vi "POST (Multipart).vi"(6 "timeout":i32=10000, 7 "output file":path, 8 "error in":errorcluster, 9 "data":T1[](array[typedef]), 10 "url":string, 11 "Session In":refnum<class "Session.lvclass">) -> (0 "error out":errorcluster, 1 "body":string, 2 "headers":string, 3 "Session Out":refnum<class "Session.lvclass">, 4 "status code":u32)   [LabVIEW 2020, in "Library Commun.lvlib" / "Library Http.lvlib" / "Session.lvclass"]
uses:
  Session.lvclass
  Multipart Data--cluster.ctl
  Session.lvclass/Session.ctl
  lvwebclient_32.dll
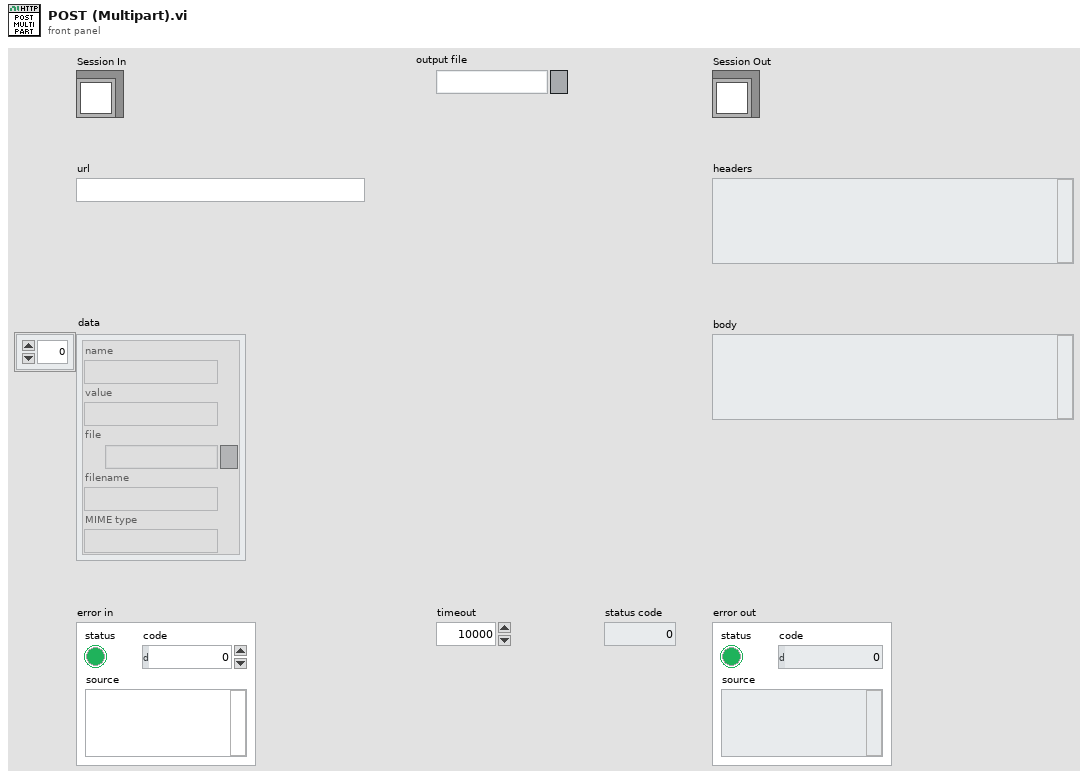
[diagram p1: front panel]
types:
  T1 = typedef "Library Commun.lvlib/Library Http.lvlib/Session.lvclass/Multipart Data--cluster.ctl" = cluster{"name":string, "value":string, "file":path, "filename":string, "MIME type":string}
  T2 = cluster{"utf-8 text":string, "utf-8 text":string, "file":path, "utf-8 text":string, "utf-8 text":string}
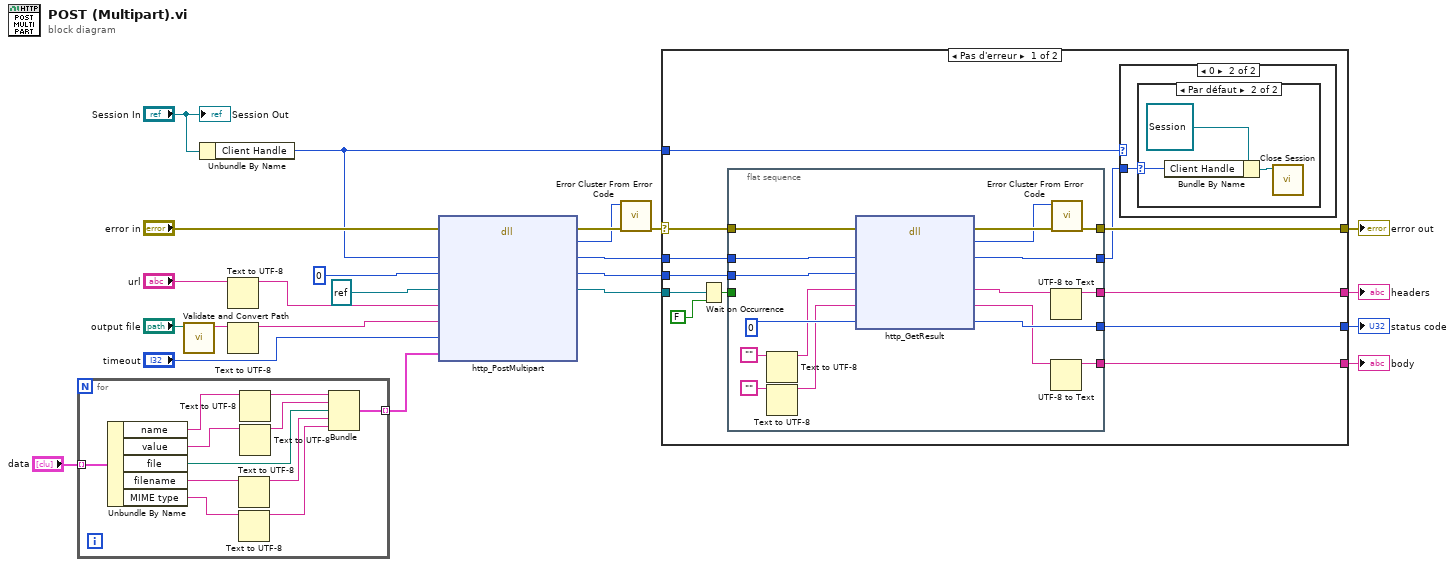
[diagram p0: block diagram]
diagram:
  n1 = for {
    tunnel: "data" -> [w34] mode=indexing
    tunnel: [w24] -> w1 mode=indexing
    n2 = Unbundle By Name(w34) -> ("name"=w33:string, "value"=w32:string, "file"=w29:path, "filename"=w28:string, "MIME type"=w26:string)
    n3 = Text to UTF-8(11:w28) -> (3:w27:string)  [unwired: 2 in, 1 out]
    n4 = Text to UTF-8(11:w26) -> (3:w25:string)  [unwired: 2 in, 1 out]
    n5 = Text to UTF-8(11:w33) -> (3:w31:string)  [unwired: 2 in, 1 out]
    n6 = Text to UTF-8(11:w32) -> (3:w30:string)  [unwired: 2 in, 1 out]
    n7 = Bundle("utf-8 text"=w31, "utf-8 text"=w30, "file"=w29, "utf-8 text"=w27, "utf-8 text"=w25) -> (w24:T2)  [unwired: 1 in]
  }
  n8 = call "Validate and Convert Path.vi"("path"="output file") -> ("validated path as string"=w15:string)  [unwired: 10 in]
  n9 = Unbundle By Name("Session In") -> ("Client Handle"=w11:u32)
  n10 = Text to UTF-8(11:"url") -> (3:w5:string)  [unwired: 2 in, 1 out]
  n11 = Text to UTF-8(11:w15) -> (3:w4:string)  [unwired: 2 in, 1 out]
  n12 = dll-call lib="C:/Users/ngarcin/OneDrive - Altyor/Standard TB/Class/Http Altyor/lvwebclient_*.*" fn="http_PostMultipart"(error in="error in", "handle"=w11, "request"=u32 0, "completeOccurrence"=refnum<k4> refnum ("occurrence"), "url"=w5, "outPath"=w4, "timeout"="timeout", "postData"=w1) -> (error out=w13:errorcluster, "return"=w12:i32, "handle"=w9:u32, "request"=w8:u32, "completeOccurrence"=w6:refnum<k4>)  [unwired: 6 in, 1 out]
  n13 = call <vilib>:"Error Cluster From Error Code.vi"("error in (no error)"=w13, "error code (0)"=w12) -> ("error out"=w23:errorcluster)  [unwired: 7 in]
  n14 = case shown="Pas d'erreur" w23 {
    selector: w23 -> [w44 w68]
    tunnel: w6 -> [w46 _]
    tunnel: w9 -> [w43 _]
    tunnel: w8 -> [w42 _]
    tunnel: [w41 _] -> w20
    tunnel: [w40 _] -> w19
    tunnel: [w39 _] -> w18
    tunnel: [w38 w68] -> w17
    tunnel: w11 -> [w37 _]
    frame No Error {
      n15 = Wait on Occurrence(1:FALSE, 2:w46) -> (0:w45:bool)  [unwired: 1 in]
      n16 = flat-sequence {
        tunnel: w45 -> [_]
        tunnel: w44 -> [w67]
        tunnel: w43 -> [w66]
        tunnel: w42 -> [w65]
        tunnel: [w63] -> w41
        tunnel: [w58] -> w40
        tunnel: [w57] -> w39
        tunnel: [w56] -> w38
        tunnel: [w55] -> w36
        frame #0 {
          n17 = Text to UTF-8(11:"") -> (3:w52:string)  [unwired: 2 in, 1 out]
          n18 = Text to UTF-8(11:"") -> (3:w51:string)  [unwired: 2 in, 1 out]
          n19 = dll-call lib="C:/Users/ngarcin/OneDrive - Altyor/Standard TB/Class/Http Altyor/lvwebclient_*.*" fn="http_GetResult"(error in=w67, "handle"=w66, "request"=w65, "returnHeader"=w52, "returnBody"=w51, "httpStatus"=u32 0) -> (error out=w62:errorcluster, "return"=w61:i32, "handle"=w55:u32, "returnHeader"=w60:string, "returnBody"=w59:string, "httpStatus"=w63:u32)  [unwired: 3 in, 1 out]
          n20 = UTF-8 to Text(11:w60) -> (3:w58:string)  [unwired: 2 in, 1 out]
          n21 = UTF-8 to Text(11:w59) -> (3:w57:string)  [unwired: 2 in, 1 out]
          n22 = call <vilib>:"Error Cluster From Error Code.vi"("error in (no error)"=w62, "error code (0)"=w61) -> ("error out"=w56:errorcluster)  [unwired: 7 in]
        }
      }
      n23 = case shown="0" w37 {
        tunnel: w36 -> [_ w47]
        frame Default {
        }
        frame 0 {
          n24 = case shown="Par défaut" w47 {
            selector: w47 -> [_ w50]
            frame 0 {
            }
            frame Default {
              n25 = Bundle By Name(cluster=refnum<class "Session.lvclass"> refnum ("NI_Advanced HTTP Client.lvlib:Session.lvclass"), "Client Handle"=w50) -> (w49:refnum<class "Session.lvclass">)
              n26 = call "Close Session.vi"("Session In"=w49) -> ()  [unwired: 10 in, 1 out]
            }
          }
        }
      }
    }
    frame Error {
    }
  }
  "error out" <- w17
  "headers" <- w19
  "body" <- w18
  "status code" <- w20
  "Session Out" <- "Session In"
